vi "Create Analog Input Vrms Module.vi"(8 "error in":errorcluster, 10 "channel settings":T1[](array[typedef]), 11 "module in":refnum<class "Module.lvclass">) -> (0 "error out":errorcluster, 3 "module out":refnum<class "Module.lvclass">)   [LabVIEW 2017, in "Scan Engine Scripting.lvlib" / "Module.lvclass"]
uses:
  Module.lvclass
  Mode Classes/Controls/analog channel settings.ctl
  Mode Classes/Analog Input Vrms Mode/Analog Input Vrms Mode.lvclass
  C:/Users/nitest/Documents/niveristand-scan-engine-ethercat-custom-device/Custom Device Source/Scripting/Modules/Mode Classes/Mode/Mode.lvclass
  C:/Users/nitest/Documents/niveristand-scan-engine-ethercat-custom-device/Custom Device Source/Scripting/Modules/Mode Classes/Analog Input Mode/Analog Input Vrms Mode/Analog Input Mode.lvclass
  Channel Classes/AI Channel/AI Channel.lvclass
  C:/Users/nitest/Documents/niveristand-scan-engine-ethercat-custom-device/Custom Device Source/Scripting/Modules/Channel Classes/Channel/Channel.lvclass
  Mode Classes/Analog Input Mode/Analog Input Vrms Mode/Analog Input Mode.lvclass
  Scan Engine Scripting.lvlib
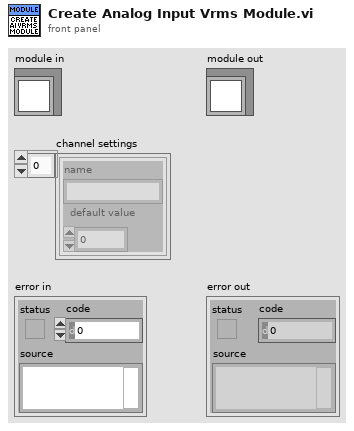
[diagram p1: front panel]
types:
  T1 = typedef "Scan Engine Scripting.lvlib/analog channel settings.ctl" = cluster{"name":string, "default value":dbl}
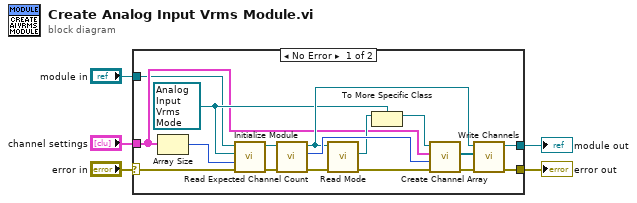
[diagram p0: block diagram]
diagram:
  n1 = case shown="No Error" "error in" {
    selector: "error in" -> [w9 w24]
    tunnel: [w8 w24] -> w4
    tunnel: [w6 w23] -> w2
    tunnel: "module in" -> [w7 w23]
    tunnel: "channel settings" -> [w10 _]
    frame No Error {
      w12 = refnum<class "Analog Input Vrms Mode.lvclass"> refnum ("Scan Engine Scripting.lvlib:Analog Input Vrms Mode.lvclass")
      n2 = Array Size(array=w10) -> (size(s)=w17:i32)
      n3 = call-dynamic "Initialize Module.vi"("error in"=w9, "channel array size"=w17, "mode"=w12, "module in"=w7) -> ("error out"=w21:errorcluster, "module out"=w22:refnum<class "Module.lvclass">)  [unwired: 6 in]
      n4 = call-dynamic "Read Expected Channel Count.vi"("error in"=w21, "module in"=w22) -> ("error out"=w14:errorcluster, "expected channel count"=w18:i32, "module out"=w16:refnum<class "Module.lvclass">)  [unwired: 7 in]
      n5 = call-dynamic "Read Mode.vi"("error in"=w14, "module in"=w16) -> ("error out"=w15:errorcluster, "mode"=w13:refnum<class "Mode.lvclass">)  [unwired: 7 in, 1 out]
      n6 = To More Specific Class(target class=w12, reference=w13) -> (specific class reference=w11:refnum<class "Analog Input Vrms Mode.lvclass">)  [unwired: 1 in, 1 out]
      n7 = call "Create Channel Array.vi"("error in"=w15, "expected channel count"=w18, "channel settings"=w10, "analog input mode in"=w11) -> ("error out"=w20:errorcluster, "channels"=w19:refnum<class "AI Channel.lvclass">[])  [unwired: 5 in, 1 out]
      n8 = call-dynamic "Write Channels.vi"("error in"=w20, "channels"=w19, "module in"=w16) -> ("error out"=w8:errorcluster, "module out"=w6:refnum<class "Module.lvclass">)  [unwired: 7 in]
    }
    frame Error {
    }
  }
  "error out" <- w4
  "module out" <- w2
